vi "Configure OVP.vi"(7 "Enable OVP (T:Enable)":bool=TRUE, 8 "error in (no error)":errorcluster, 9 "Voltage Unit(V)":u16(ring) items=["V", "mV", "kV"], 10 "Voltage Limit(0.0V)":dbl format="%_2g", 11 "VISA resource name":refnum<visa-resource-name>) -> (0 "error out":errorcluster, 3 "VISA resource name out":refnum<visa-resource-name>)   [LabVIEW 2013, in "Keithley 2200 Series.lvlib"]
doc: "Configure OVP and Send Over Voltage limit to power supply."
uses:
  Keithley 2200 Series.lvlib
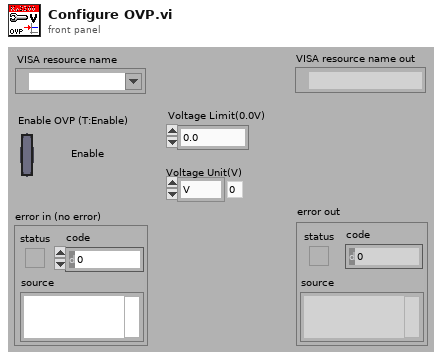
[diagram p1: front panel]
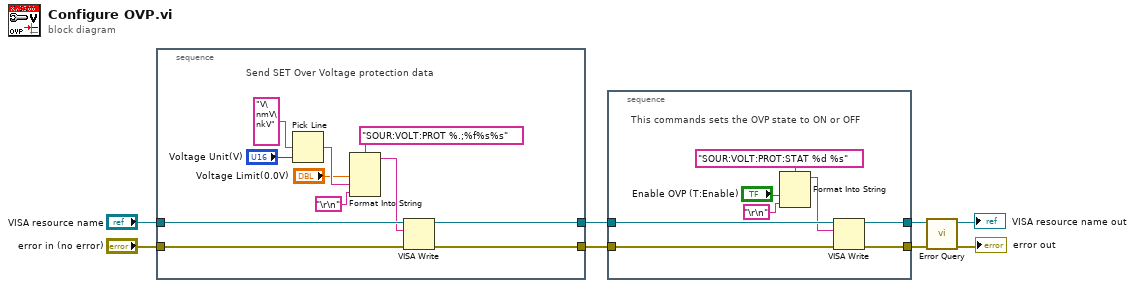
[diagram p0: block diagram]
diagram:
  n1 = stacked-sequence {
    tunnel: [w13] -> w4
    tunnel: [w12] -> w3
    tunnel: "VISA resource name" -> [w11]
    tunnel: "error in (no error)" -> [w10]
    frame #0 {
      # "Send SET Over Voltage protection data"
      n2 = Pick Line(multi-line string="V\nmV\nkV", line index="Voltage Unit(V)") -> (output string=w18:string)  [unwired: 1 out]
      n3 = Format Into String(format string="SOUR:VOLT:PROT %.;%f%s%s", "Voltage Limit(0.0V)", w18, "\r\n") -> (resulting string=w9:string)  [unwired: 2 in, 1 out]
      n4 = VISA Write(VISA resource name=w11, write buffer=w9, error in (no error)=w10) -> (VISA resource name out=w13:refnum<visa-resource-name>, error out=w12:errorcluster)  [unwired: 1 out]
    }
  }
  n5 = stacked-sequence {
    tunnel: w4 -> [w25]
    tunnel: w3 -> [w24]
    tunnel: [w23] -> w2
    tunnel: [w22] -> w1
    frame #0 {
      # "This commands sets the OVP state to ON or OFF"
      n6 = Format Into String(format string="SOUR:VOLT:PROT:STAT %d %s", "Enable OVP (T:Enable)", "\r\n") -> (resulting string=w20:string)  [unwired: 2 in, 1 out]
      n7 = VISA Write(VISA resource name=w25, write buffer=w20, error in (no error)=w24) -> (VISA resource name out=w23:refnum<visa-resource-name>, error out=w22:errorcluster)  [unwired: 1 out]
    }
  }
  n8 = call "Error Query.vi"("error in (no error)"=w1, "VISA resource name"=w2) -> ("error out"=→"error out":errorcluster, "VISA resource name out"=→"VISA resource name out":refnum<visa-resource-name>)  [unwired: 8 out]
